vi "FTW-Ether-Address-Validate.vi"(5 "Address":string, 11 "error in":errorcluster) -> (6 "Sanitized Address":string, 8 "Message Transport Scheme":T1, 15 "error out":errorcluster)   [LabVIEW 2013, in "FTW-Ether.lvclass"]
uses:
  FTW-Ether.lvclass
  FTW-Ether-MessageTransportScheme.ctl
panel:
  # "Inputs"
  # "Outputs"
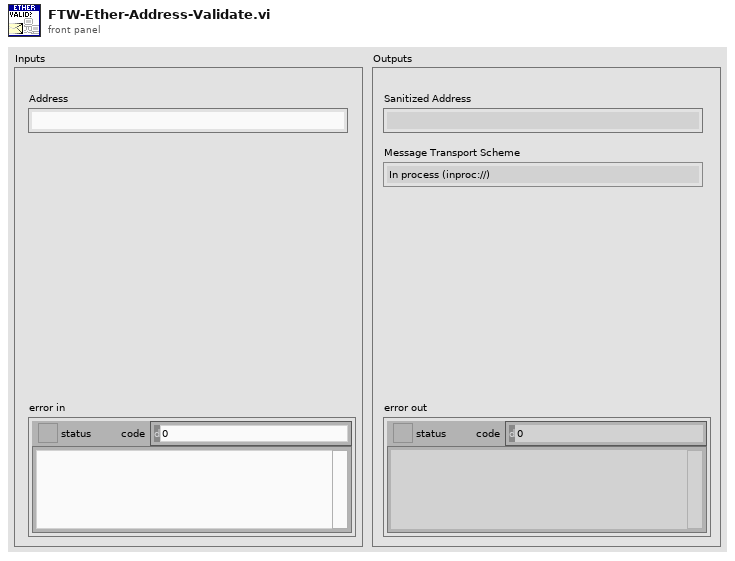
[diagram p1: front panel]
types:
  T1 = typedef "FTW-Ether.lvclass/FTW-Ether-MessageTransportScheme.ctl" = enum16{"In process (inproc://)", "TCP (tcp://)"}
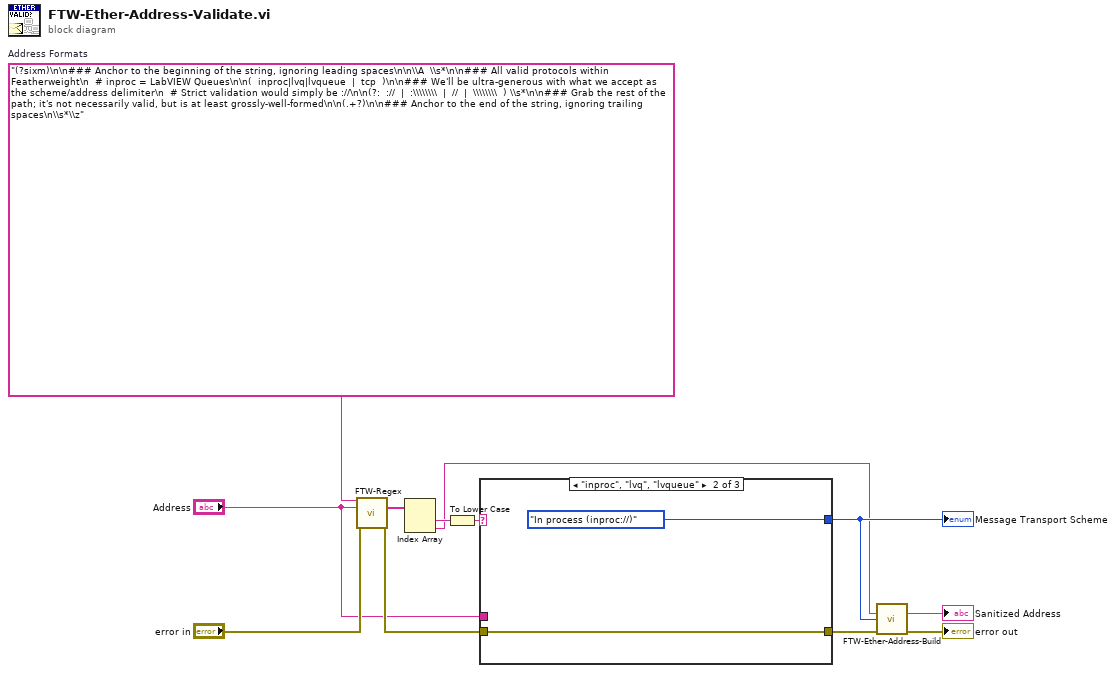
[diagram p0: block diagram]
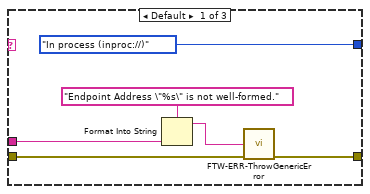
[diagram p2: hidden frame]
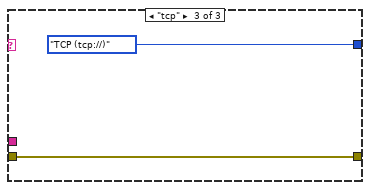
[diagram p3: hidden frame]
diagram:
  w12 = "(?sixm)\n\n### Anchor to the beginning of the string, ignoring leading spaces\n\n\\A  \\s*\n\n### All valid protocols within Featherweight\n  # inproc = LabVIEW Queues\n\n(  inproc|lvq|lvqueue  |  tcp  )\n\n### We'll be ultra-generous with what we accept as the scheme/address delimiter\n  # Strict validation would simply be ://\n\n(?:  ://  |  :\\\\\\\\  |  //  |  \\\\\\\\  ) \\s*\n\n### Grab the rest of the path; it's not necessarily valid, but is at least grossly-well-formed\n\n(.+?)\n\n### Anchor to the end of the string, ignoring trailing spaces\n\\s*\\z"  # Address Formats
  n1 = call "FTW-Regex.vi"("Regular Expression"=w12, "Input String"="Address", "error in"="error in") -> ("Submatches"=w11:string[], "error out"=w7:errorcluster)  [unwired: 8 in, 3 out]
  n2 = Index Array(array=w11) -> (element #1=w9:string, element #2=w1:string)  [unwired: 2 in]
  n3 = To Lower Case(string=w9) -> (all lower case string=w8:string)
  n4 = case shown="\"inproc\", \"lvq\", \"lvqueue\"" w8 {
    tunnel: [FTW-Ether-MessageTransportScheme."In process (inproc://)" ("Message Transport Scheme") FTW-Ether-MessageTransportScheme."In process (inproc://)" ("Message Transport Scheme") FTW-Ether-MessageTransportScheme."TCP (tcp://)" ("Message Transport Scheme")] -> w2
    tunnel: w7 -> [w15 w19 w21]
    tunnel: "Address" -> [w14 _ _]
    tunnel: [w13 w19 w21] -> w3
    frame Default {
      n5 = Format Into String(format string="Endpoint Address \"%s\" is not well-formed." ("Error Message"), w14) -> (resulting string=w17:string)  [unwired: 2 in, 1 out]
      n6 = call "FTW-ERR-ThrowGenericError.vi"("Error Message"=w17, "error in"=w15) -> ("error out"=w13:errorcluster)  [unwired: 13 in]
    }
    frame "inproc", "lvq", "lvqueue" {
    }
    frame "tcp" {
    }
  }
  "Message Transport Scheme" <- w2
  n7 = call "FTW-Ether-Address-Build.vi"("Path"=w1, "Message Transport Scheme"=w2, "error in"=w3) -> ("Endpoint Address"=→"Sanitized Address":string, "error out"=→"error out":errorcluster)  [unwired: 11 in]
